vi "wait_milliseconds.vi"(9 "milliseconds to wait":u32, 11 "error in":errorcluster) -> (3 "error out":errorcluster)   [LabVIEW 2018]
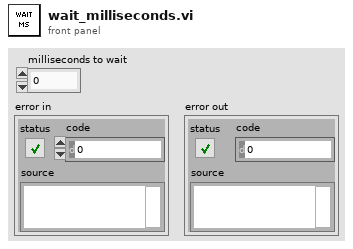
[diagram p1: front panel]
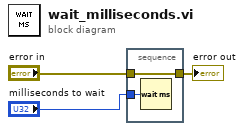
[diagram p0: block diagram]
diagram:
  n1 = stacked-sequence {
    tunnel: "error in" -> [w5]
    tunnel: [w5] -> w2
    tunnel: "milliseconds to wait" -> [w4]
    frame #0 {
      n2 = Wait (ms)(milliseconds to wait=w4) -> ()  [unwired: 1 out]
    }
  }
  "error out" <- w2
